vi "步响应V0.vi"(3 "NbOfPointsToAverage":dbl=1000.0, 4 "X_value_end":dbl, 5 "行程 in":dbl[](array[numeric])) -> (1 "V0":dbl, 2 "行程 out":dbl[](array[numeric]))   [LabVIEW 2013]
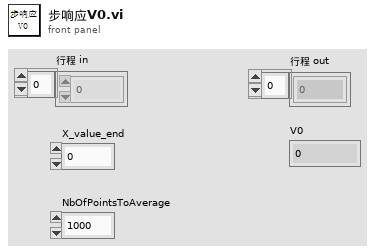
[diagram p1: front panel]
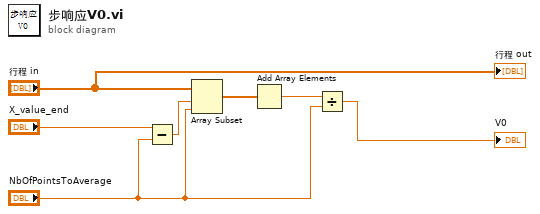
[diagram p0: block diagram]
diagram:
  n1 = Subtract(x="X_value_end", y="NbOfPointsToAverage") -> (x-y=w5:dbl)
  n2 = Array Subset(array="行程 in", index=w5, length="NbOfPointsToAverage") -> (w7:dbl[])
  n3 = Add Array Elements(numeric array=w7) -> (sum=w6:dbl)
  n4 = Divide(x=w6, y="NbOfPointsToAverage") -> (x/y=→"V0":dbl)
  "行程 out" <- "行程 in"
